vi "7.2.3 Joystick Mapping.vi"(1 "button info":T2, 2 "axis info":T3, 3 "Saitek Controler 3":T1 {"Right" scale=-32767.0..32767.0; "Left" scale=-32767.0..32767.0; "Yaw" scale=-32767.0..32767.0; "Roll" scale=-32767.0..32767.0; "Pitch" scale=-32767.0..32767.0}) -> (0 "Saitek Controler 2":T1 {"Right" scale=-32767.0..32767.0; "Left" scale=-32767.0..32767.0; "Yaw" scale=-32767.0..32767.0; "Roll" scale=-32767.0..32767.0; "Pitch" scale=-32767.0..32767.0})   [LabVIEW 2010]
uses:
  6-OCU Neurons/6.1-UDP Saitek.ctl
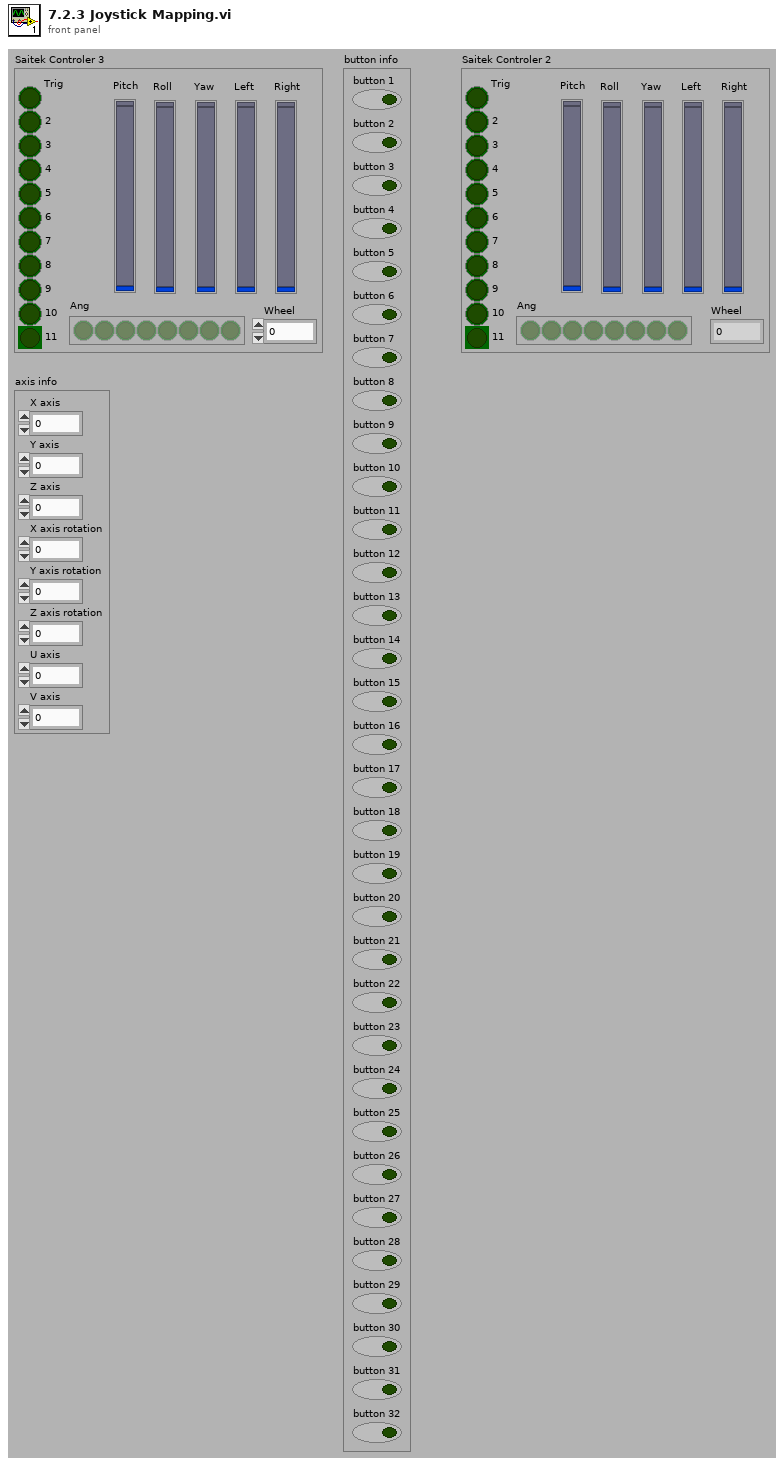
[diagram p1: front panel]
types:
  T1 = typedef "6.1-UDP Saitek.ctl" = cluster{"Trig":bool, "2":bool, "3":bool, "4":bool, "5":bool, "6":bool, "7":bool, "8":bool, "9":bool, "10":bool, "11":bool, "Pitch":i32, "Ang":bool[], "Wheel":dbl, "Roll":i32, "Yaw":i32, "Left":i32, "Right":i32}
  T2 = cluster{"button 1":bool, "button 2":bool, "button 3":bool, "button 4":bool, "button 5":bool, "button 6":bool, "button 7":bool, "button 8":bool, "button 9":bool, "button 10":bool, "button 11":bool, "button 12":bool, "button 13":bool, "button 14":bool, "button 15":bool, "button 16":bool, "button 17":bool, "button 18":bool, "button 19":bool, "button 20":bool, "button 21":bool, "button 22":bool, "button 23":bool, "button 24":bool, "button 25":bool, "button 26":bool, "button 27":bool, "button 28":bool, "button 29":bool, "button 30":bool, "button 31":bool, "button 32":bool}
  T3 = cluster{"X axis":i32, "Y axis":i32, "Z axis":i32, "X axis rotation":i32, "Y axis rotation":i32, "Z axis rotation":i32, "U axis":i32, "V axis":i32}
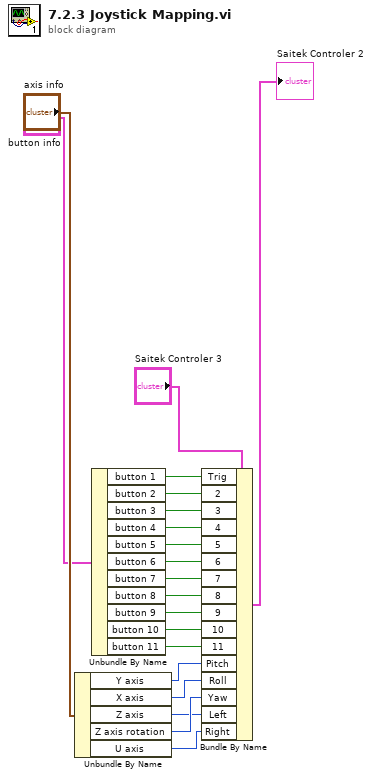
[diagram p0: block diagram]
diagram:
  n1 = Unbundle By Name("axis info") -> ("Y axis"=w20:i32, "X axis"=w18:i32, "Z axis"=w16:i32, "Z axis rotation"=w19:i32, "U axis"=w17:i32)
  n2 = Unbundle By Name("button info") -> ("button 1"=w13:bool, "button 2"=w12:bool, "button 3"=w11:bool, "button 4"=w10:bool, "button 5"=w9:bool, "button 6"=w8:bool, "button 7"=w7:bool, "button 8"=w6:bool, "button 9"=w5:bool, "button 10"=w4:bool, "button 11"=w3:bool)
  n3 = Bundle By Name(cluster="Saitek Controler 3", "Trig"=w13, "2"=w12, "3"=w11, "4"=w10, "5"=w9, "6"=w8, "7"=w7, "8"=w6, "9"=w5, "10"=w4, "11"=w3, "Pitch"=w20, "Roll"=w18, "Yaw"=w19, "Left"=w16, "Right"=w17) -> (→"Saitek Controler 2":T1)
